vi "TCP Writer.vi"(1 "occurrence":refnum<k4>, 2 "DeviceType for TCP":T1) -> (0 "stopped":bool)   [LabVIEW 2020]
uses:
  Shared/TCP/DeviceType-enum.ctl
  Device Drivers/shared/stop FGV control.ctl
panel:
  in  "error in":errorcluster
  out "time for sending TCP":u32(graph)
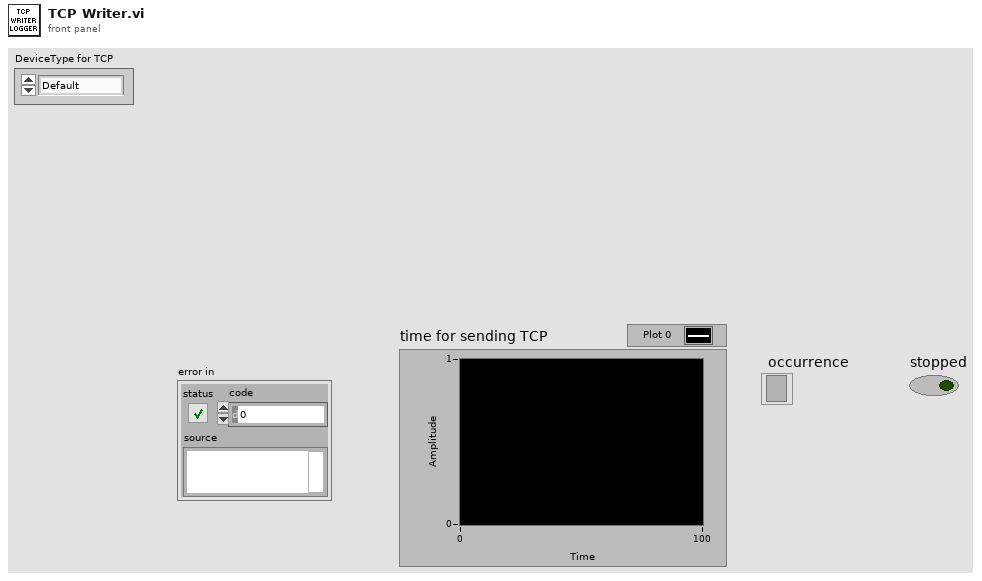
[diagram p1: front panel]
types:
  T1 = typedef "DeviceType-enum.ctl" = enum16{"Default", "Logger"}
  T2 = typedef "stop FGV control.ctl" = enum16{"Clear", "Write", "Read"}
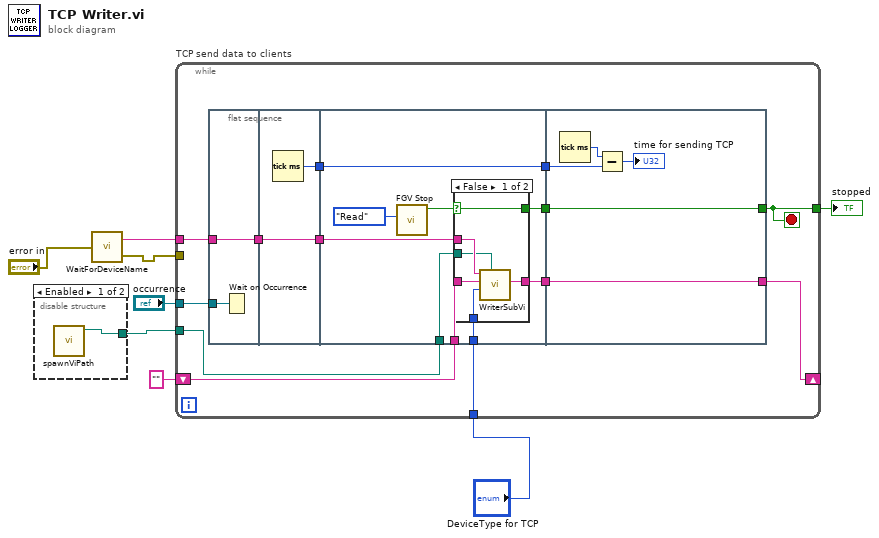
[diagram p0: block diagram]
diagram:
  n1 = disable-structure shown="Enabled" {
    disable-tunnel: [w9 _] -> w8
    frame Enabled {
      n2 = call "spawnViPath.vi"() -> ("Spawn vi path"=w9:path)  [unwired: 10 in, 1 out]
    }
    frame Disabled {
    }
  }
  n3 = call "WaitForDeviceName.vi"("error in 2"="error in") -> ("Device Name"=w6:string, "error in"=w5:errorcluster)
  n4 = while "TCP send data to clients" {
    tunnel: "occurrence" -> [w22]
    tunnel: [w21] -> w3
    tunnel: w5 -> [_]
    tunnel: w6 -> [w20]
    shift-right: [w19] -> _
    shift-left: "" ("head buffer out") -> [w18]
    tunnel: w8 -> [w11]
    tunnel: "DeviceType for TCP" -> [w10]
    stop <- w21 stop-if-true
    n5 = flat-sequence {
      tunnel: w22 -> [w24]
      tunnel: w20 -> [w23]
      tunnel: [w23] -> w17
      tunnel: w17 -> [w26]
      tunnel: [w26] -> w16
      tunnel: [w25] -> w13
      tunnel: w16 -> [w33]
      tunnel: w18 -> [w31]
      tunnel: [w34] -> w15
      tunnel: [w32] -> w14
      tunnel: w13 -> [w30]
      tunnel: [w30] -> w12
      tunnel: w11 -> [w29]
      tunnel: w10 -> [w27]
      tunnel: [w47] -> w19
      tunnel: [w48] -> w21
      tunnel: w15 -> [w48]
      tunnel: w14 -> [w47]
      tunnel: w12 -> [w45]
      frame #0 {
        n6 = Wait on Occurrence(2:w24) -> ()  [unwired: 2 in, 1 out]
      }
      frame #1 {
        n7 = Tick Count (ms)() -> (millisecond timer value=w25:u32)
      }
      frame #2 {
        n8 = call "FGV Stop.vi"("Function"=stop_FGV_control."Read") -> ("stop out"=w35:bool)  [unwired: 9 in, 1 out]
        n9 = case shown="False" w35 {
          selector: w35 -> [w41 w43]
          tunnel: [w41 w43] -> w34
          tunnel: w33 -> [w40 _]
          tunnel: [w39 w42] -> w32
          tunnel: w31 -> [w38 w42]
          tunnel: w29 -> [w37 _]
          tunnel: w27 -> [w36 _]
          frame False {
            n10 = call "WriterSubVi.vi"("Spawn vi path"=w37, "DeviceType for TCP"=w36, "head buffer"=w38, "Device Name"=w40) -> ("head buffer out"=w39:string)  [unwired: 6 in, 1 out]
          }
          frame True {
          }
        }
      }
      frame #3 {
        n11 = Tick Count (ms)() -> (millisecond timer value=w46:u32)
        n12 = Subtract(x=w46, y=w45) -> (x-y=→"time for sending TCP":u32)
      }
    }
  }
  "stopped" <- w3
